vi "AD_DA_trig.vi"() -> ()   [LabVIEW 2012]
uses:
  <vilib>/Utility/error.llb/DialogType.ctl
  <vilib>/DAQmx/read.llb/DAQmx Read (Analog DBL 1Chan 1Samp).vi
  <vilib>/DAQmx/write.llb/DAQmx Write (Analog 1D Wfm NChan NSamp).vi
  <vilib>/DAQmx/create/channels.llb/DAQmx Create Channel (AI-Voltage-Basic).vi
  <vilib>/DAQmx/configure/timing.llb/DAQmx Timing (Sample Clock).vi
  <vilib>/DAQmx/configure/task.llb/DAQmx Configure Logging (TDMS).vi
  <vilib>/DAQmx/create/channels.llb/DAQmx Create Channel (AO-Voltage-Basic).vi
  <vilib>/DAQmx/configure/trigger.llb/DAQmx Start Trigger (Digital Edge).vi
  <vilib>/DAQmx/configure/trigger.llb/DAQmx Start Trigger (Analog Edge).vi
  <vilib>/DAQmx/miscellaneous.llb/DAQmx Fill In Error Info.vi
  <resource>/objmgr/daqmx.rc
panel:
  in  "Offset":dbl=4.975
  out "Waveform Graph 2":dynamicdata(graph)
  in  "Trigger Type 2":T1(tab)
  in  "Edge 2":i32(ring)=10280 items=["Rising"=10280, "Falling"=10171]
  in  "Digital Trigger Source 2":tag
  in  "Level (V) 2":dbl format="%0.2f"
  in  "Hysteresis (V) 2":dbl
  in  "Slope 2":i32(ring)=10280 items=["Rising"=10280, "Falling"=10171]
  in  "Analog Trigger Source 2":string="APFI0"
  in  "Pause When":i32(ring)=10192 items=["High"=10192, "Low"=10214]
  in  "Pause Trigger Source":tag
  in  "Sample Rate 2":dbl=1000.0
  in  "Sample Clock Source 2":tag="OnboardClock"
  in  "Max Voltage 2":dbl=5.0
  in  "Min Voltage 2":dbl=-5.0
  in  "Physical Channel(s)":tag="Dev1/ao0"
  out "Actual Sample Rate 2":dbl=1000.0 format="%0.2f"
  out "Array":dbl[](array[numeric])
  in  "Logging Mode":i32(ring)=10231 items=["Off"=10231, "Log and Read"=15842]
  out "Actual Sample Rate":dbl=1000.0 format="%0.2f"
  in  "Physical Channel":tag="Dev1/ai0"
  in  "Min Voltage":dbl=-10.0
  in  "Max Voltage":dbl=10.0
  in  "Terminal Configuration":i32(ring)=-1 items=["default"=-1, "RSE"=10083, "NRSE"=10078, "Differential"=10106, "Pseudodifferential"=12529]
  in  "Sample Clock Source":tag="OnboardClock"
  in  "Sample Rate":dbl=1000.0
  in  "TDMS File Path":path
  in  "Trigger Type":T2(tab)
  in  "Edge":i32(ring)=10280 items=["Rising"=10280, "Falling"=10171]
  in  "Digital Trigger Source":tag
  in  "Level (V)":dbl format="%0.2f"
  in  "Hysteresis (V)":dbl
  in  "Slope":i32(ring)=10280 items=["Rising"=10280, "Falling"=10171]
  in  "Analog Trigger Source":string="APFI0"
  # "To configure and use a start trigger you must have the necessary tab selected above.  Not all hardware supports triggering--refer to your device documentation for more info."
  # "To configure and use a start trigger you must have the necessary tab selected above.  Not all hardware supports triggering--refer to your device documentation for more info."
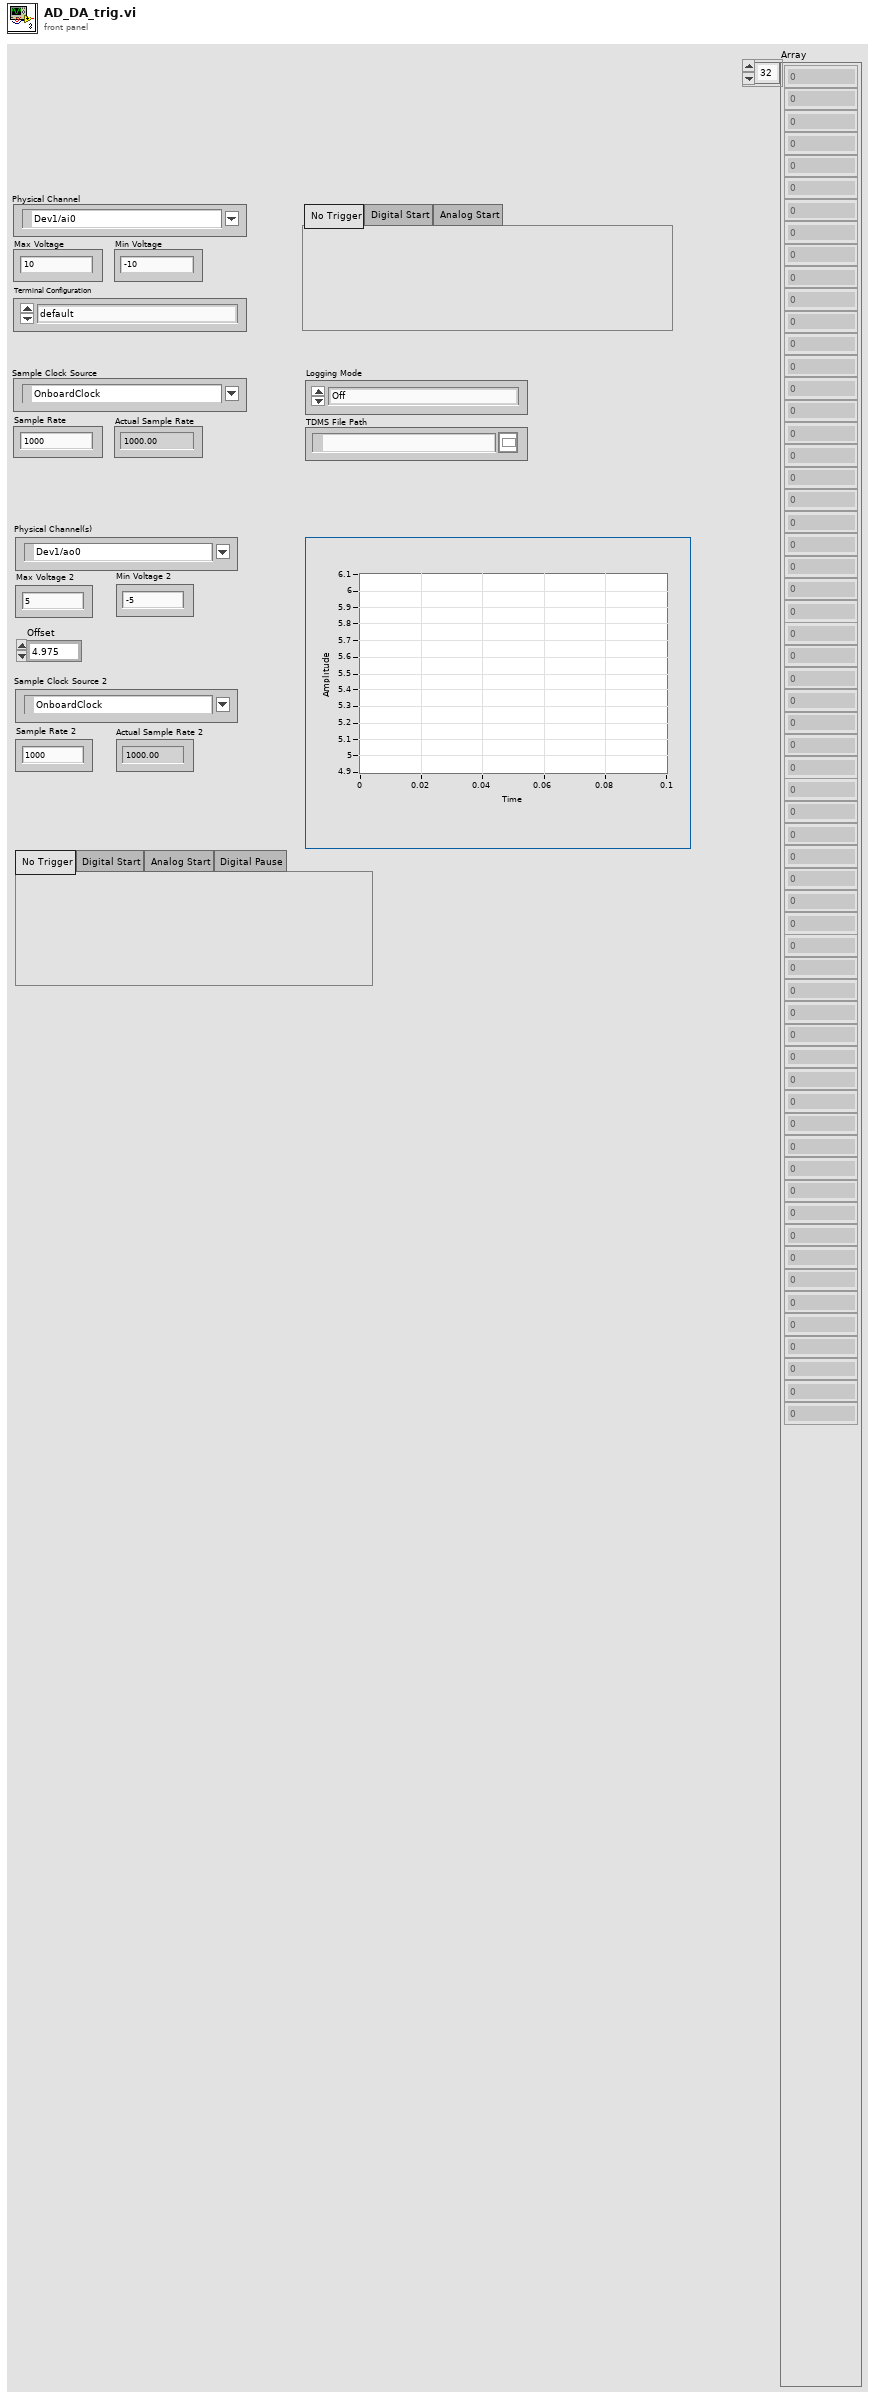
[diagram p1: front panel]
types:
  T1 = enum32{"No Trigger", "Digital Start", "Analog Start", "Digital Pause"}
  T2 = enum32{"No Trigger", "Digital Start", "Analog Start"}
  T3 = typedef "DialogType.ctl" = u16
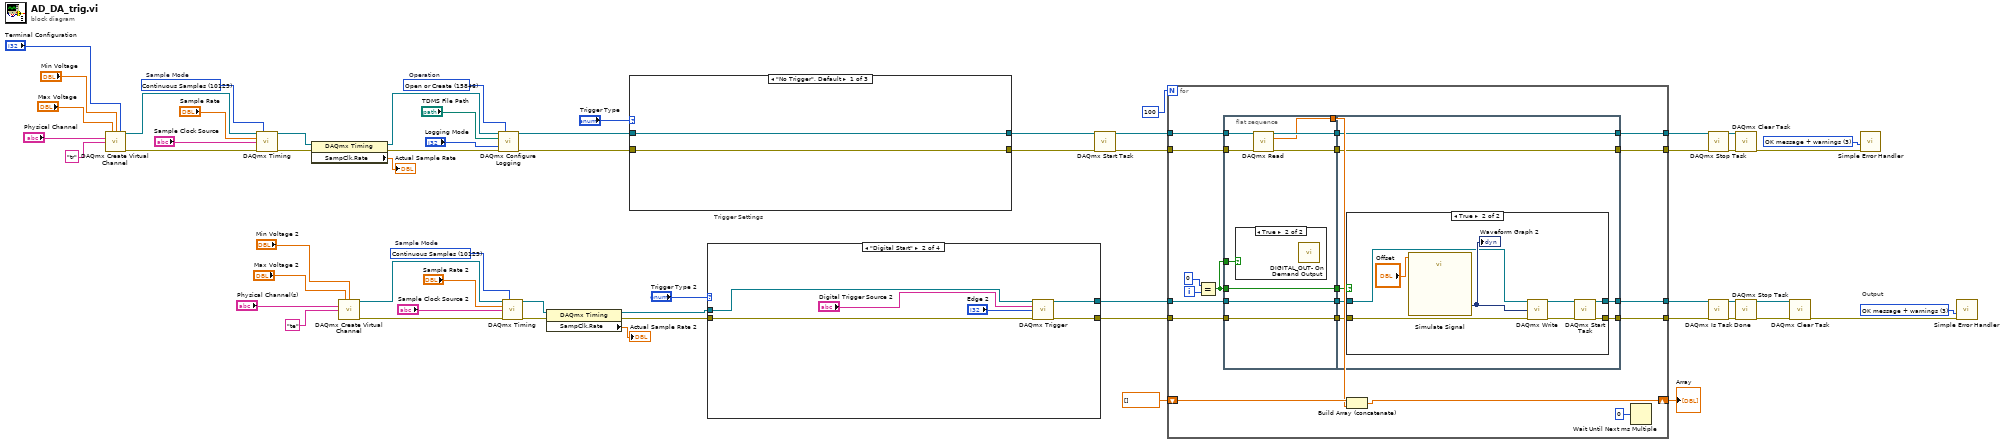
[diagram p0: block diagram]
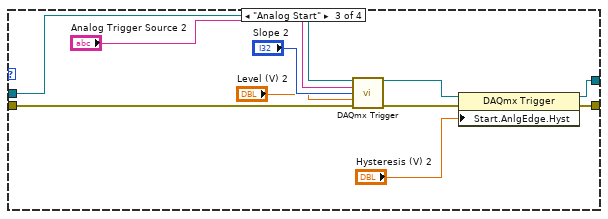
[diagram p3: hidden frame]
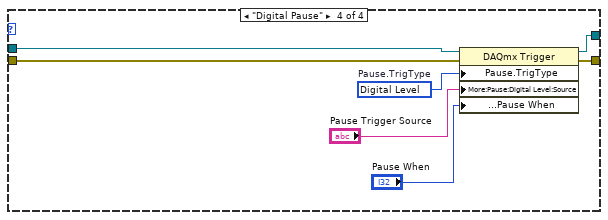
[diagram p4: hidden frame]
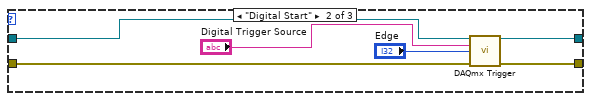
[diagram p5: hidden frame]
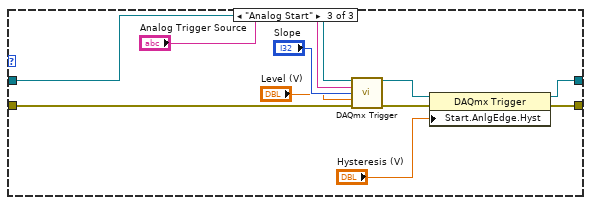
[diagram p6: hidden frame]
diagram:
  w25 = T3 3 items=["no dialog", "OK message", "continue or stop message", "OK message + warnings", "continue/stop + warnings"] ("type of dialog (OK msg:1)")
  w10 = 10123 items=["Finite Samples"=10178, "Continuous Samples"=10123, "Hardware Timed Single Point"=12522]  # Sample Mode
  w29 = T3 3 items=["no dialog", "OK message", "continue or stop message", "OK message + warnings", "continue/stop + warnings"] ("type of dialog (OK msg:1)")
  w45 = 15846 items=["Open"=10437, "Open or Create"=15846, "Create or Replace"=15847, "Create"=15848]  # Operation
  w40 = 10123 items=["Finite Samples"=10178, "Continuous Samples"=10123, "Hardware Timed Single Point"=12522]  # Sample Mode
  # "Output"
  # "Trigger Settings"
  n1 = call-poly <vilib>:"DAQmx Create Virtual Channel.vi"("maximum value"="Max Voltage", "minimum value"="Min Voltage", "input terminal configuration"="Terminal Configuration", "physical channels"="Physical Channel", "name to assign"="tr") -> ("task out"=w42:refnum<k21>, "error out"=w41:errorcluster)  [unwired: 9 in]
  n2 = call-poly <vilib>:"DAQmx Timing.vi"("task/channels in"=w42, "sample mode"=w40, "rate"="Sample Rate", "source"="Sample Clock Source", "error in"=w41) -> ("task out"=w38:refnum<k21>, "error out"=w39:errorcluster)  [unwired: 9 in]
  n3 = property class="DAQmx Timing"(reference=w38, error in=w39) -> (reference out=w43:refnum<k21>, error out=w44:errorcluster, "SampClk.Rate"=→"Actual Sample Rate":dbl)
  n4 = call-poly <vilib>:"DAQmx Create Virtual Channel.vi"("maximum value"="Max Voltage 2", "minimum value"="Min Voltage 2", "physical channels"="Physical Channel(s)", "name to assign"="te") -> ("task out"=w12:refnum<k21>, "error out"=w11:errorcluster)  [unwired: 10 in]
  n5 = call-poly <vilib>:"DAQmx Configure Logging.vi"("task/channels in"=w43, "operation"=w45, "file path"="TDMS File Path", "logging mode"="Logging Mode", "error in"=w44) -> ("task out"=w46:refnum<k21>, "error out"=w47:errorcluster)  [unwired: 9 in]
  n6 = call-poly <vilib>:"DAQmx Timing.vi"("task/channels in"=w12, "sample mode"=w10, "rate"="Sample Rate 2", "source"="Sample Clock Source 2", "error in"=w11) -> ("task out"=w8:refnum<k21>, "error out"=w9:errorcluster)  [unwired: 9 in]
  n7 = property class="DAQmx Timing"(reference=w8, error in=w9) -> (reference out=w20:refnum<k21>, error out=w21:errorcluster, "SampClk.Rate"=→"Actual Sample Rate 2":dbl)
  n8 = case shown="\"No Trigger\", Default" "Trigger Type" {
    tunnel: w46 -> [w61 w67 w77]
    tunnel: w47 -> [w60 w66 w76]
    tunnel: [w61 w65 w74] -> w48
    tunnel: [w60 w64 w73] -> w49
    frame "No Trigger", Default {
    }
    frame "Digital Start" {
      n9 = call-poly <vilib>:"DAQmx Trigger.vi"("task/channels in"=w67, "source"="Digital Trigger Source", "edge"="Edge", "error in"=w66) -> ("task out"=w65:refnum<k21>, "error out"=w64:errorcluster)  [unwired: 10 in]
    }
    frame "Analog Start" {
      n10 = call-poly <vilib>:"DAQmx Trigger.vi"("task/channels in"=w77, "source"="Analog Trigger Source", "slope"="Slope", "level"="Level (V)", "error in"=w76) -> ("task out"=w72:refnum<k21>, "error out"=w71:errorcluster)  [unwired: 9 in]
      n11 = property class="DAQmx Trigger"(reference=w72, error in=w71, "Start.AnlgEdge.Hyst"="Hysteresis (V)") -> (reference out=w74:refnum<k21>, error out=w73:errorcluster)
    }
  }
  n12 = case shown="\"Digital Start\"" "Trigger Type 2" {
    tunnel: w20 -> [w79 w85 w95 w102]
    tunnel: w21 -> [w78 w84 w94 w99]
    tunnel: [w79 w83 w92 w101] -> w4
    tunnel: [w78 w82 w91 w100] -> w3
    frame "No Trigger", Default {
    }
    frame "Digital Start" {
      n13 = call-poly <vilib>:"DAQmx Trigger.vi"("task/channels in"=w85, "source"="Digital Trigger Source 2", "edge"="Edge 2", "error in"=w84) -> ("task out"=w83:refnum<k21>, "error out"=w82:errorcluster)  [unwired: 10 in]
    }
    frame "Analog Start" {
      n14 = call-poly <vilib>:"DAQmx Trigger.vi"("task/channels in"=w95, "source"="Analog Trigger Source 2", "slope"="Slope 2", "level"="Level (V) 2", "error in"=w94) -> ("task out"=w90:refnum<k21>, "error out"=w89:errorcluster)  [unwired: 9 in]
      n15 = property class="DAQmx Trigger"(reference=w90, error in=w89, "Start.AnlgEdge.Hyst"="Hysteresis (V) 2") -> (reference out=w92:refnum<k21>, error out=w91:errorcluster)
    }
    frame "Digital Pause" {
      w98 = 10152 items=["Analog Level"=10101, "Analog Window"=10103, "Digital Level"=10152, "Digital Pattern"=10398, "None"=10230]  # Pause.TrigType
      n16 = property class="DAQmx Trigger"(reference=w102, error in=w99, "Pause.TrigType"=w98, "More:Pause:Digital Level:Source"="Pause Trigger Source", "More:Pause:Digital Level:Pause When"="Pause When") -> (reference out=w101:refnum<k21>, error out=w100:errorcluster)
    }
  }
  n17 = call <vilib>:"DAQmx Start Task.vi"("task/channels in"=w48, "error in"=w49) -> ("task out"=w35:refnum<k21>, "error out"=w33:errorcluster)  [unwired: 12 in]
  n18 = for {
    N: 100 -> [_]
    tunnel: w35 -> [w121]
    tunnel: [w120] -> w34
    tunnel: w33 -> [w119]
    tunnel: [w118] -> w32
    shift-right: [w116] -> w26
    shift-left: dbl[] [] -> [w117]
    tunnel: w4 -> [w112]
    tunnel: w3 -> [w109]
    tunnel: [w108] -> w2
    tunnel: [w107] -> w1
    i -> [w106]
    n19 = Equal?(x=0, y=w106) -> (x = y?=w103:bool)
    n20 = flat-sequence {
      tunnel: w121 -> [w131]
      tunnel: w119 -> [w129]
      tunnel: [w127] -> w115
      tunnel: [w130] -> w114
      tunnel: [w128] -> w113
      tunnel: w112 -> [w126]
      tunnel: [w126] -> w111
      tunnel: [w125] -> w110
      tunnel: w109 -> [w125]
      tunnel: w103 -> [w124]
      tunnel: [w123] -> w104
      tunnel: w103 -> [w123]
      tunnel: [w137] -> w118
      tunnel: [w138] -> w120
      tunnel: w114 -> [w138]
      tunnel: w113 -> [w137]
      tunnel: w111 -> [w136]
      tunnel: w110 -> [w135]
      tunnel: [w134] -> w108
      tunnel: [w133] -> w107
      tunnel: w104 -> [w132]
      frame #0 {
        n21 = case shown="True" w124 {
          frame False {
          }
          frame True {
            n22 = call "DIGITAL_OUT- On Demand Output.vi"() -> ()  [unwired: 12 in]
          }
        }
        n23 = call-poly <vilib>:"DAQmx Read.vi"("task/channels in"=w131, "error in"=w129) -> ("task out"=w130:refnum<k21>, "data"=w127:dbl, "error out"=w128:errorcluster)  [unwired: 11 in]
      }
      frame #1 {
        n24 = case shown="True" w132 {
          tunnel: w136 -> [w140 w144]
          tunnel: w135 -> [w139 w143]
          tunnel: [w140 w142] -> w134
          tunnel: [w139 w141] -> w133
          frame False {
          }
          frame True {
            n25 = call "Simulate Signal"("Offset"="Offset") -> ("DC"=w146:dynamicdata)  [unwired: 13 in, 1 out]
            "Waveform Graph 2" <- w146
            n26 = call-poly <vilib>:"DAQmx Write.vi"("task/channels in"=w144, "data"=w146, "error in"=w143) -> ("task out"=w148:refnum<k21>, "error out"=w147:errorcluster)  [unwired: 10 in, 1 out]
            n27 = call <vilib>:"DAQmx Start Task.vi"("task/channels in"=w148, "error in"=w147) -> ("task out"=w142:refnum<k21>, "error out"=w141:errorcluster)  [unwired: 12 in]
          }
        }
      }
    }
    n28 = Build Array (concatenate)(w117, w115) -> (w116:dbl[])
    n29 = Wait Until Next ms Multiple(millisecond multiple=u32 0) -> ()  [unwired: 1 out]
  }
  "Array" <- w26
  n30 = call <vilib>:"DAQmx Stop Task.vi"("task/channels in"=w34, "error in"=w32) -> ("task out"=w37:refnum<k21>, "error out"=w36:errorcluster)  [unwired: 12 in]
  n31 = call <vilib>:"DAQmx Is Task Done.vi"("task/channels in"=w2, "error in"=w1) -> ("task out"=w6:refnum<k21>, "error out"=w5:errorcluster)  [unwired: 11 in, 1 out]
  n32 = call <vilib>:"DAQmx Clear Task.vi"("task in"=w37, "error in"=w36) -> ("error out"=w30:errorcluster)  [unwired: 13 in]
  n33 = call <vilib>:"DAQmx Stop Task.vi"("task/channels in"=w6, "error in"=w5) -> ("task out"=w23:refnum<k21>, "error out"=w24:errorcluster)  [unwired: 12 in]
  n34 = call <vilib>:"DAQmx Clear Task.vi"("task in"=w23, "error in"=w24) -> ("error out"=w13:errorcluster)  [unwired: 13 in]
  n35 = call <vilib>:"Simple Error Handler.vi"("type of dialog (OK msg:1)"=w29, "error in (no error)"=w30) -> ()  [unwired: 3 in, 5 out]
  n36 = call <vilib>:"Simple Error Handler.vi"("type of dialog (OK msg:1)"=w25, "error in (no error)"=w13) -> ()  [unwired: 3 in, 5 out]
